vi "Identify.vi"(8 "error in (no error)":errorcluster, 11 "PSU in":refnum<class "Simulated Power Supply.lvclass">) -> (0 "error out":errorcluster, 2 "Identification":string, 3 "PSU out":refnum<class "Simulated Power Supply.lvclass">)   [LabVIEW 2017, in "Power Supply Driver.lvlib" / "Simulated Power Supply.lvclass"]
uses:
  Simulated Power Supply.lvclass
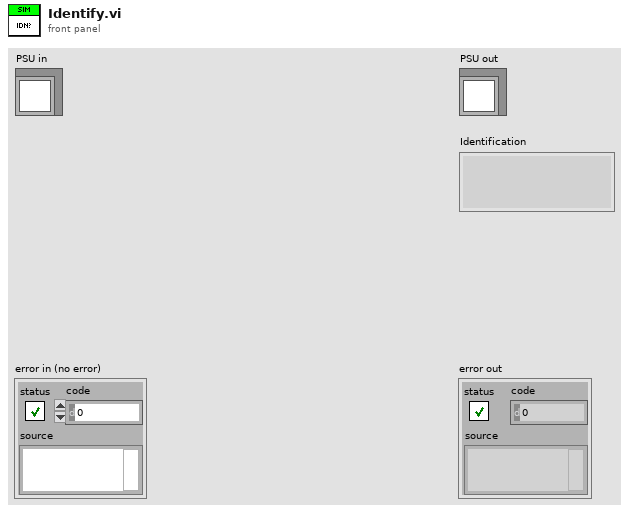
[diagram p1: front panel]
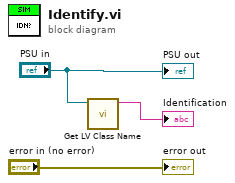
[diagram p0: block diagram]
diagram:
  n1 = call <vilib>:"Get LV Class Name.vi"("object"="PSU in") -> ("class name"=→"Identification":string)  [unwired: 9 in, 1 out]
  "error out" <- "error in (no error)"
  "PSU out" <- "PSU in"
